vi "load_xml.vi"(8 "error in":errorcluster, 10 "child node in":refnum<k20>, 11 "Hamamatsu_C9100-13.lvclass (in)":refnum<class "Hamamatsu_C9100-13.lvclass">) -> (0 "error out":errorcluster, 2 "child node out":refnum<k20>, 3 "Hamamatsu_C9100-13.lvclass":refnum<class "Hamamatsu_C9100-13.lvclass">)   [LabVIEW 2014, in "Hamamatsu_C9100-13.lvclass"]
doc: "Loads Hamamatsu C9100-13 camera settings from xml. Expected format:\n\n<Enable>%b</Enable>\n<AnalogGain>%u</AnalogGain>\n<FrameGrabberAcquisitionRegion columns=\"left, top, right, bottom\">%u %u %u %u</FrameGrabberAcquisitionRegion>\n<ExposureTime>%f</ExposureTime>\n<EMGain>%u</EMGain>\n<TriggerPolarity>%s</TriggerPolarity>\n<ExternalTriggerMode>%s</ExternalTriggerMode>\n<ScanSpeed>%s</ScanSpeed>\n<ExternalTriggerSource>%s</ExternalTriggerSource>\n<ScanMode>%s</ScanMode>\n<SuperPixelBinning>%s</SuperPixelBinning>\n<CameraSubArrayAcquisitionRegion columns=\"left, top, width, height\">%u %u %u %u</CameraSubArrayAcquisitionRegion>\n<NumberOfImageBuffers>%u</NumberOfImageBuffers>\n<RegionsOfInterest columns=\"Left, Top, Right Bottom\">\n%s</RegionsOfInterest>\n<BackgroundRegions columns=\"Left, Top, Right Bottom\">\n%s</BackgroundRegions>\n<ShotsPerMeasurement>%u</ShotsPerMeasurement>\n<PhotoelectronScaling>%f</PhotoelectronScaling>\n\nMTL 2013 Jan 1"
uses:
  Hamamatsu_C9100-13.lvclass
  Hamamatsu_C9100-13.lvclass/Hamamatsu_C9100-13.ctl
  Globals.vi
  <vilib>/xml/Close Reference(Node).vi
  <resource>/objmgr/DOMUserDefRef.rc
  <vilib>/xml/NI_XML.lvlib
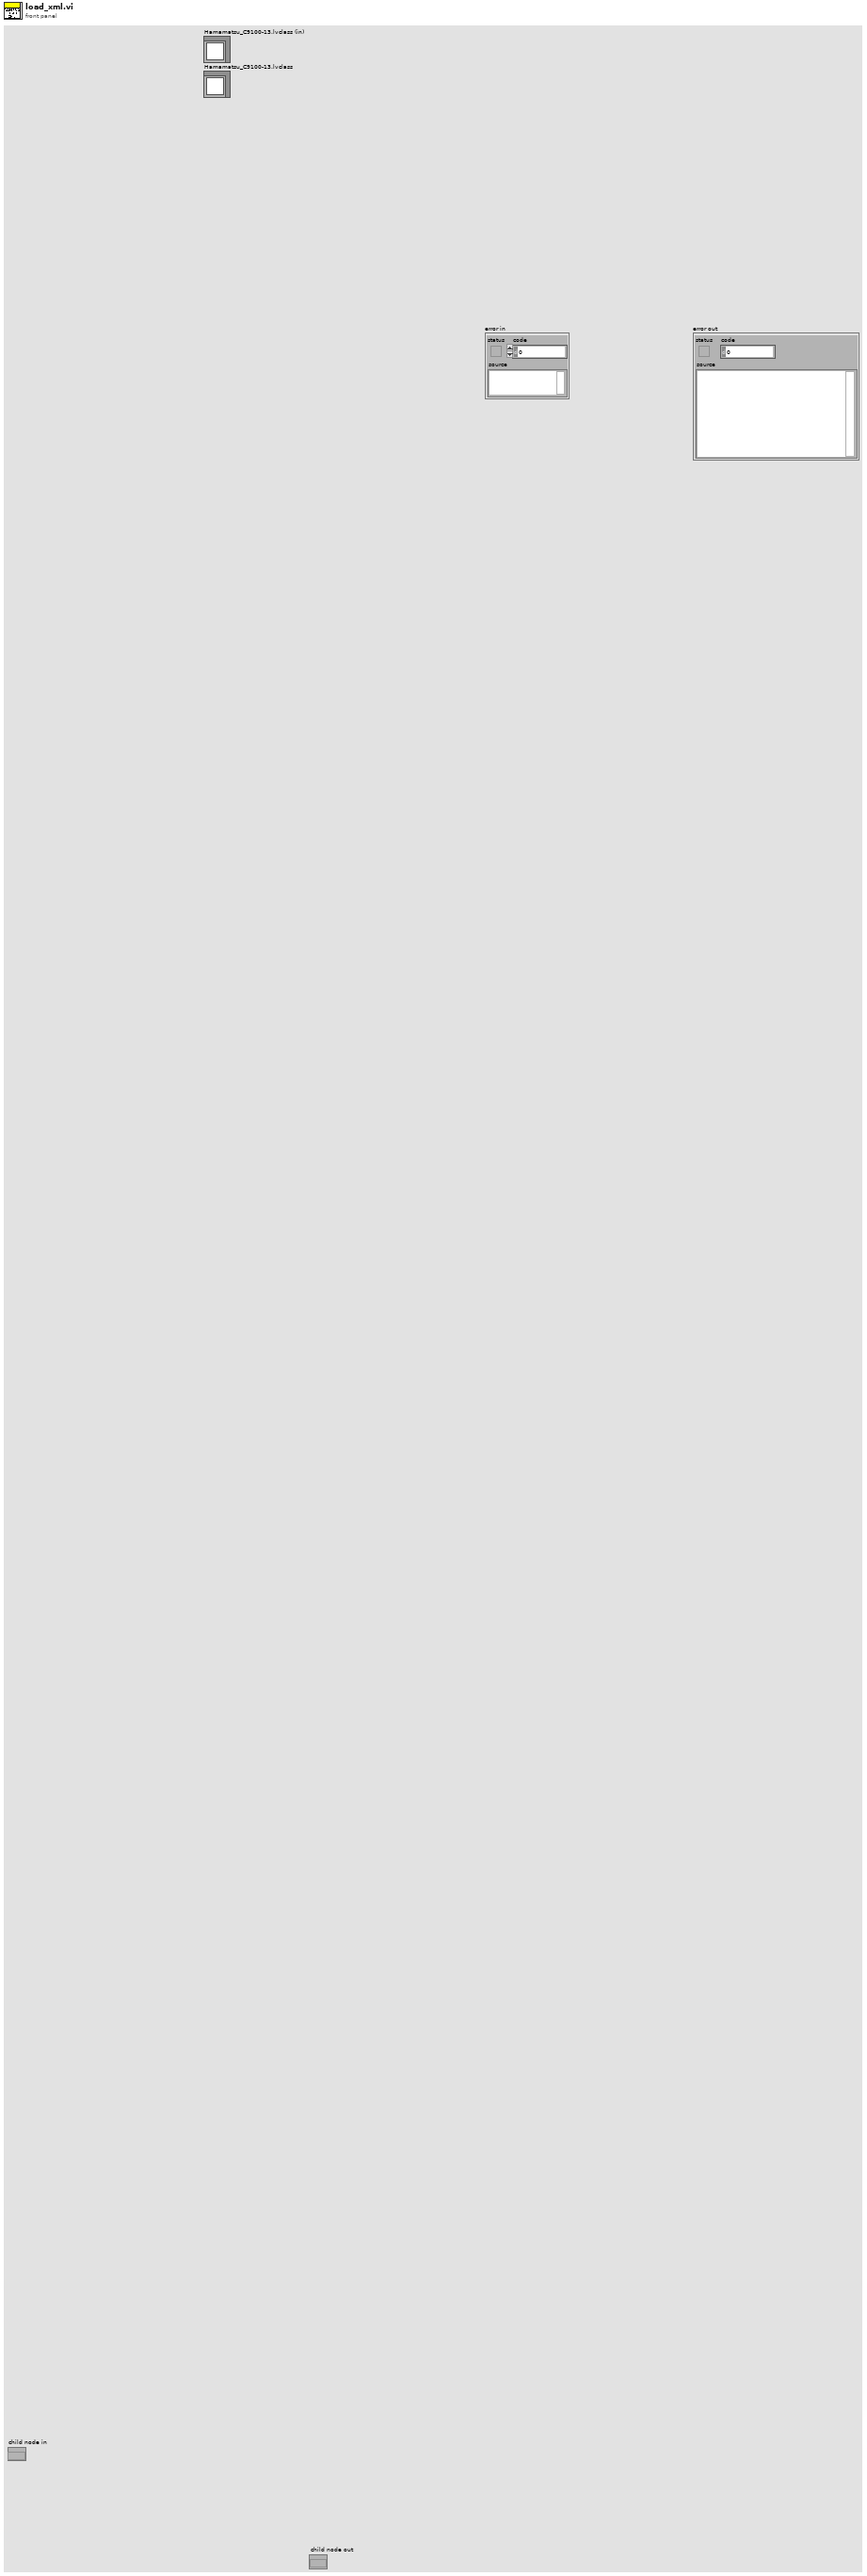
[diagram p1: front panel]
types:
  T1 = typedef "Hamamatsu_C9100-13.lvclass/camera_setup.ctl" = cluster{"Analog Gain (0-5)":u8, "Exposure Time":dbl, "EM Gain (0-255)":u8, "Trigger Polarity":string, "External Trigger Mode":string, "Scan Speed":string, "External Trigger Source":string, "Scan Mode":string, "Super Pixel Binning\n(if enabled in Scan Mode)":string, "Camera Sub-array acquisition region\n(if enabled in scan mode)":cluster{"Left":u16, "Top":u16, "Width":u16, "Height":u16}, "Use camera?":bool, "# image buffers":i32, "shots per measurement":i32, "Force images to U16":bool, "Low Light Sensitivity":string, "cooling":string, "fan":string, "Frame Grabber acquisition region":cluster{"Left":i32, "Top":i32, "Right":i32, "Bottom":i32}}
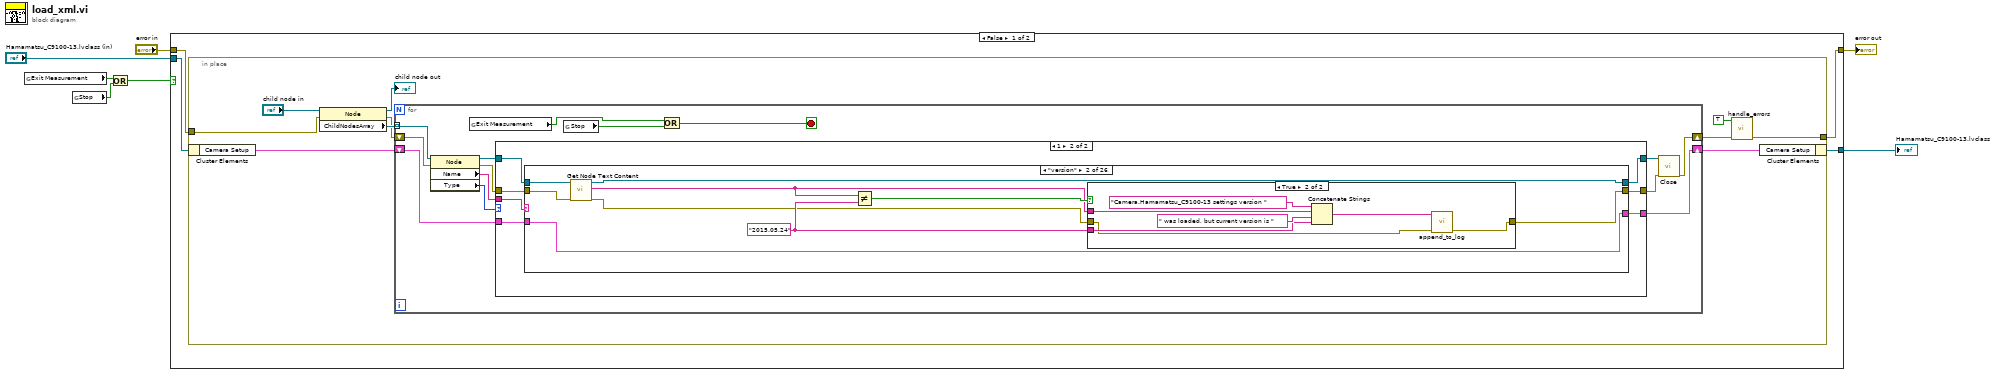
[diagram p0: block diagram]
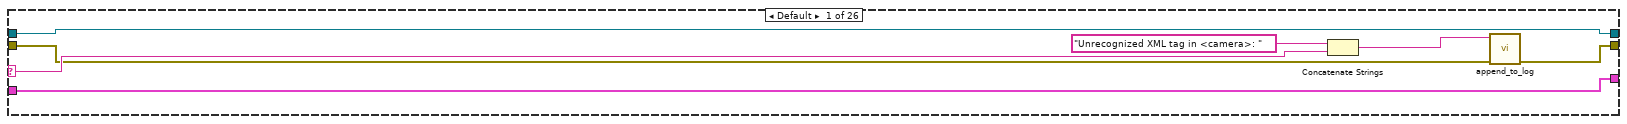
[diagram p3: hidden frame]
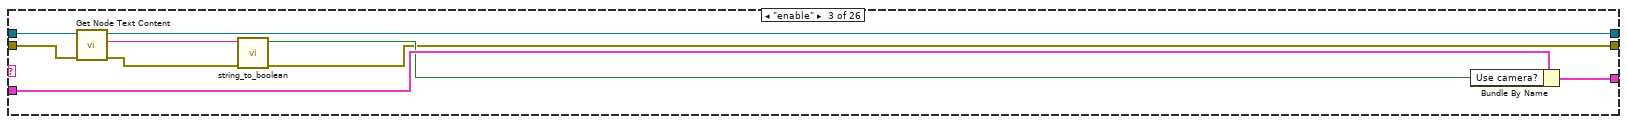
[diagram p5: hidden frame]
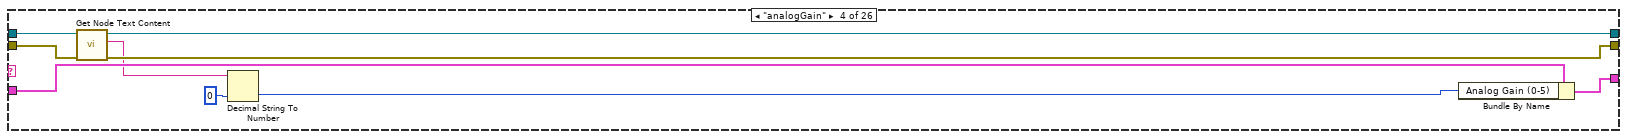
[diagram p6: hidden frame]
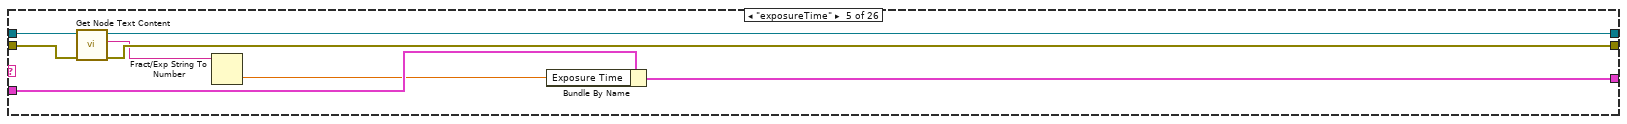
[diagram p7: hidden frame]
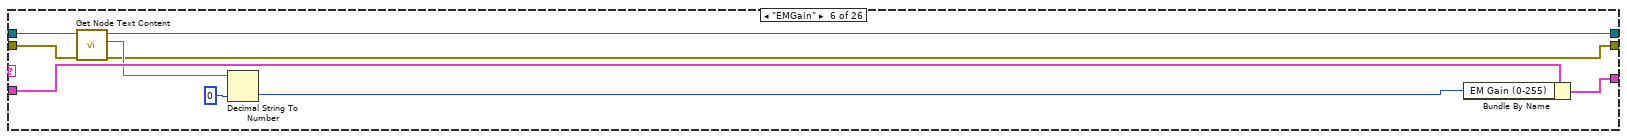
[diagram p8: hidden frame]
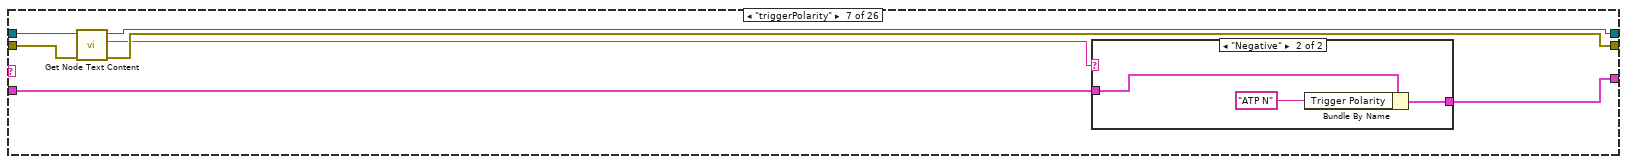
[diagram p9: hidden frame]
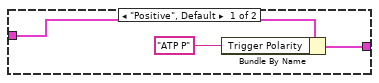
[diagram p10: hidden frame]
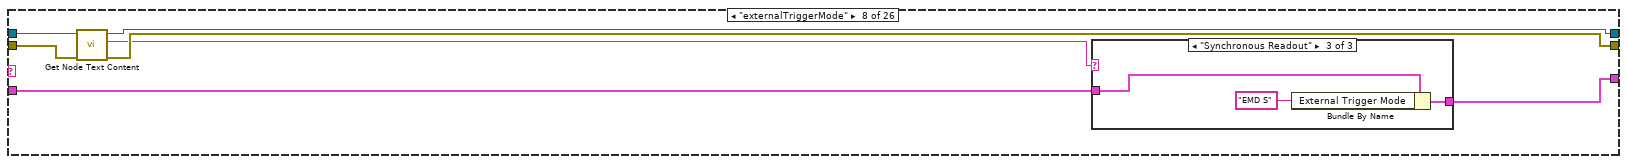
[diagram p11: hidden frame]
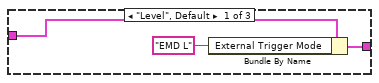
[diagram p12: hidden frame]
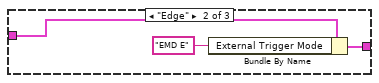
[diagram p13: hidden frame]
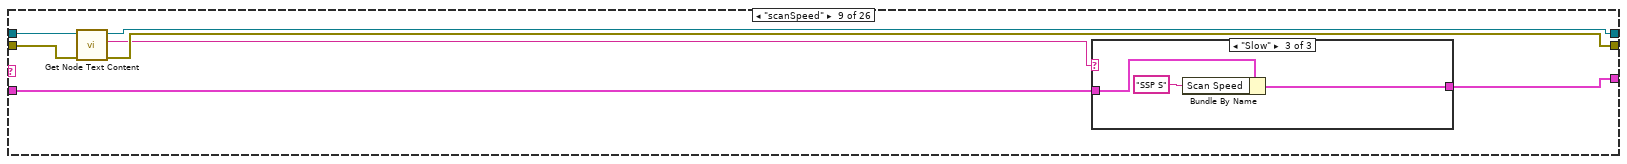
[diagram p14: hidden frame]
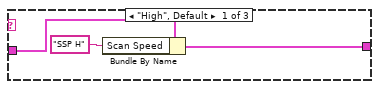
[diagram p15: hidden frame]
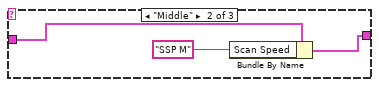
[diagram p16: hidden frame]
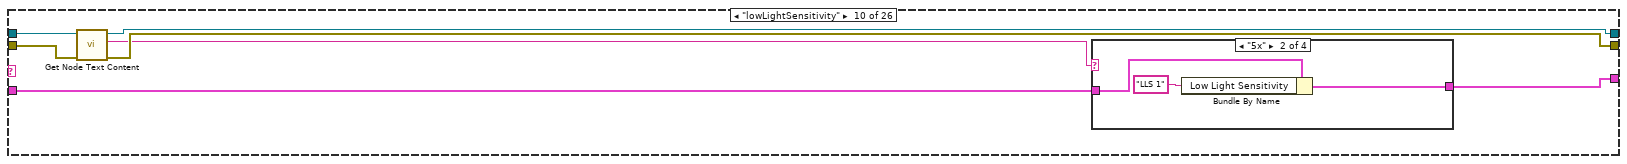
[diagram p17: hidden frame]
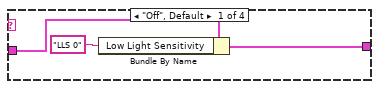
[diagram p18: hidden frame]
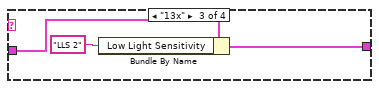
[diagram p19: hidden frame]
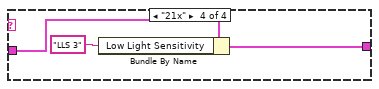
[diagram p20: hidden frame]
diagram:
  n1 = global read "Globals.vi" "Exit Measurement"() -> (w6:bool)
  n2 = global read "Globals.vi" "Stop"() -> (w5:bool)
  n3 = Or(x=w6, y=w5) -> (x .or. y?=w4:bool)
  n4 = case shown="False" w4 {
    tunnel: [w8 w334] -> w7
    tunnel: "error in" -> [w11 w334]
    tunnel: "Hamamatsu_C9100-13.lvclass (in)" -> [w10 w333]
    tunnel: [w9 w333] -> w1
    frame False {
      n5 = in-place {
        in-place-border: [w16] -> w8
        in-place-border: w11 -> [w15]
        n6 = in-place-cluster #1(w10) -> ("Camera Setup"=w13:T1)
        n7 = property class="Node"(reference="child node in", error in=w15) -> (reference out=→"child node out":refnum<k20>, error out=w19:errorcluster, "ChildNodesArray"=w21:refnum<k20>[])
        n8 = for {
          tunnel: w21 -> [w26] mode=indexing
          shift-right: [w32] -> w14
          shift-left: w13 -> [w33]
          shift-right: [w29] -> w17
          shift-left: w19 -> [w27]
          stop <- w22 stop-if-true
          n9 = property class="Node"(reference=w26, error in=w27) -> (reference out=w34:refnum<k20>, error out=w30:errorcluster, "Name"=w35:string, "Type"=w25:i32)
          n10 = global read "Globals.vi" "Exit Measurement"() -> (w24:bool)
          n11 = case shown="1" w25 {
            tunnel: w35 -> [_ w45]
            tunnel: w34 -> [w38 w44]
            tunnel: w33 -> [w36 w43]
            tunnel: [w36 w42] -> w32
            tunnel: [w38 w41] -> w31
            tunnel: w30 -> [w37 w40]
            tunnel: [w37 w39] -> w28
            frame Default {
            }
            frame 1 {
              n12 = case shown="\"version\"" w45 {
                selector: w45 -> [w48 _ _ _ _ _ _ _ _ _ _ _ _ _ _ _ _ _ _ _ _ _ _ _ _ _]
                tunnel: w44 -> [w51 w56 w77 w84 w92 w103 w110 w123 w139 w155 w174 w190 w203 w216 w230 w241 w250 w259 w268 w277 w286 w295 w304 w313 w322 w331]
                tunnel: w43 -> [w52 w55 w75 w87 w95 w101 w107 w120 w136 w152 w171 w187 w199 w213 w233 w238 w247 w256 w265 w274 w283 w292 w301 w311 w320 w324]
                tunnel: [w52 w55 w74 w86 w94 w100 w106 w119 w135 w151 w170 w186 w198 w212 w232 w234 w243 w252 w261 w270 w279 w288 w297 w310 w319 w329] -> w42
                tunnel: [w51 w54 w78 w85 w93 w104 w111 w124 w140 w156 w175 w191 w204 w217 w231 w239 w248 w257 w266 w275 w284 w293 w302 w314 w323 w332] -> w41
                tunnel: w40 -> [w47 w57 w76 w83 w91 w102 w109 w122 w138 w154 w173 w189 w202 w215 w229 w242 w251 w260 w269 w278 w287 w296 w305 w312 w321 w330]
                tunnel: [w46 w53 w70 w82 w90 w98 w108 w121 w137 w153 w172 w188 w201 w214 w228 w240 w249 w258 w267 w276 w285 w294 w303 w308 w317 w327] -> w39
                frame Default {
                  n13 = Concatenate Strings("Unrecognized XML tag in <camera>: " ("string"), w48) -> (w49:string)
                  n14 = call "append_to_log.vi"("error in"=w47, "string"=w49) -> ("error out"=w46:errorcluster)  [unwired: 9 in]
                }
                frame "version" {
                  w59 = "2015.05.24" ("y")
                  n15 = call <vilib>:"Get Node Text Content.vi"("error in (no error)"=w57, "node in"=w56) -> ("error out"=w58:errorcluster, "node text"=w60:string, "node out"=w54:refnum<k20>)  [unwired: 7 in]
                  n16 = Not Equal?(x=w60, y=w59) -> (x != y?=w61:bool)
                  n17 = case shown="True" w61 {
                    tunnel: w60 -> [_ w68]
                    tunnel: w59 -> [_ w66]
                    tunnel: w58 -> [w62 w64]
                    tunnel: [w62 w63] -> w53
                    frame False {
                    }
                    frame True {
                      n18 = Concatenate Strings("Camera.Hamamatsu_C9100-13 settings version " ("string"), w68, " was loaded, but current version is " ("string"), w66) -> (w65:string)
                      n19 = call "append_to_log.vi"("error in"=w64, "string"=w65) -> ("error out"=w63:errorcluster)  [unwired: 9 in]
                    }
                  }
                }
                frame "enable" {
                  n20 = call <vilib>:"Get Node Text Content.vi"("error in (no error)"=w76, "node in"=w77) -> ("error out"=w72:errorcluster, "node text"=w73:string, "node out"=w78:refnum<k20>)  [unwired: 7 in]
                  n21 = call "string_to_boolean.vi"("error in"=w72, "string"=w73) -> ("error out"=w70:errorcluster, "boolean"=w71:bool)  [unwired: 8 in]
                  n22 = Bundle By Name(cluster=w75, "Use camera?"=w71) -> (w74:T1)
                }
                frame "analogGain" {
                  n23 = call <vilib>:"Get Node Text Content.vi"("error in (no error)"=w83, "node in"=w84) -> ("error out"=w82:errorcluster, "node text"=w81:string, "node out"=w85:refnum<k20>)  [unwired: 7 in]
                  n24 = Decimal String To Number(string=w81, default (0L)=u8 0 ("Analog Gain (0-5)")) -> (number=w79:u8)  [unwired: 1 in, 1 out]
                  n25 = Bundle By Name(cluster=w87, "Analog Gain (0-5)"=w79) -> (w86:T1)
                }
                frame "exposureTime" {
                  n26 = call <vilib>:"Get Node Text Content.vi"("error in (no error)"=w91, "node in"=w92) -> ("error out"=w90:errorcluster, "node text"=w89:string, "node out"=w93:refnum<k20>)  [unwired: 7 in]
                  n27 = Fract/Exp String To Number(string=w89) -> (number=w88:dbl)  [unwired: 3 in, 1 out]
                  n28 = Bundle By Name(cluster=w95, "Exposure Time"=w88) -> (w94:T1)
                }
                frame "EMGain" {
                  n29 = call <vilib>:"Get Node Text Content.vi"("error in (no error)"=w102, "node in"=w103) -> ("error out"=w98:errorcluster, "node text"=w99:string, "node out"=w104:refnum<k20>)  [unwired: 7 in]
                  n30 = Decimal String To Number(string=w99, default (0L)=u8 0 ("EM Gain (0-255)")) -> (number=w96:u8)  [unwired: 1 in, 1 out]
                  n31 = Bundle By Name(cluster=w101, "EM Gain (0-255)"=w96) -> (w100:T1)
                }
                frame "triggerPolarity" {
                  n32 = call <vilib>:"Get Node Text Content.vi"("error in (no error)"=w109, "node in"=w110) -> ("error out"=w108:errorcluster, "node text"=w105:string, "node out"=w111:refnum<k20>)  [unwired: 7 in]
                  n33 = case shown="\"Negative\"" w105 {
                    tunnel: w107 -> [w114 w117]
                    tunnel: [w113 w116] -> w106
                    frame "Positive", Default {
                      n34 = Bundle By Name(cluster=w114, "Trigger Polarity"="ATP P" ("fan")) -> (w113:T1)
                    }
                    frame "Negative" {
                      n35 = Bundle By Name(cluster=w117, "Trigger Polarity"="ATP N" ("fan")) -> (w116:T1)
                    }
                  }
                }
                frame "externalTriggerMode" {
                  n36 = call <vilib>:"Get Node Text Content.vi"("error in (no error)"=w122, "node in"=w123) -> ("error out"=w121:errorcluster, "node text"=w118:string, "node out"=w124:refnum<k20>)  [unwired: 7 in]
                  n37 = case shown="\"Synchronous Readout\"" w118 {
                    tunnel: w120 -> [w127 w130 w133]
                    tunnel: [w126 w129 w132] -> w119
                    frame "Level", Default {
                      n38 = Bundle By Name(cluster=w127, "External Trigger Mode"="EMD L" ("fan")) -> (w126:T1)
                    }
                    frame "Edge" {
                      n39 = Bundle By Name(cluster=w130, "External Trigger Mode"="EMD E" ("fan")) -> (w129:T1)
                    }
                    frame "Synchronous Readout" {
                      n40 = Bundle By Name(cluster=w133, "External Trigger Mode"="EMD S" ("fan")) -> (w132:T1)
                    }
                  }
                }
                frame "scanSpeed" {
                  n41 = call <vilib>:"Get Node Text Content.vi"("error in (no error)"=w138, "node in"=w139) -> ("error out"=w137:errorcluster, "node text"=w134:string, "node out"=w140:refnum<k20>)  [unwired: 7 in]
                  n42 = case shown="\"Slow\"" w134 {
                    tunnel: w136 -> [w143 w146 w149]
                    tunnel: [w142 w145 w148] -> w135
                    frame "High", Default {
                      n43 = Bundle By Name(cluster=w143, "Scan Speed"="SSP H" ("fan")) -> (w142:T1)
                    }
                    frame "Middle" {
                      n44 = Bundle By Name(cluster=w146, "Scan Speed"="SSP M" ("fan")) -> (w145:T1)
                    }
                    frame "Slow" {
                      n45 = Bundle By Name(cluster=w149, "Scan Speed"="SSP S" ("fan")) -> (w148:T1)
                    }
                  }
                }
                frame "lowLightSensitivity" {
                  n46 = call <vilib>:"Get Node Text Content.vi"("error in (no error)"=w154, "node in"=w155) -> ("error out"=w153:errorcluster, "node text"=w150:string, "node out"=w156:refnum<k20>)  [unwired: 7 in]
                  n47 = case shown="\"5x\"" w150 {
                    tunnel: w152 -> [w159 w162 w165 w168]
                    tunnel: [w158 w161 w164 w167] -> w151
                    frame "Off", Default {
                      n48 = Bundle By Name(cluster=w159, "Low Light Sensitivity"="LLS 0" ("fan")) -> (w158:T1)
                    }
                    frame "5x" {
                      n49 = Bundle By Name(cluster=w162, "Low Light Sensitivity"="LLS 1" ("fan")) -> (w161:T1)
                    }
                    frame "13x" {
                      n50 = Bundle By Name(cluster=w165, "Low Light Sensitivity"="LLS 2" ("fan")) -> (w164:T1)
                    }
                    frame "21x" {
                      n51 = Bundle By Name(cluster=w168, "Low Light Sensitivity"="LLS 3" ("fan")) -> (w167:T1)
                    }
                  }
                }
                frame "externalTriggerSource" {
                  n52 = call <vilib>:"Get Node Text Content.vi"("error in (no error)"=w173, "node in"=w174) -> ("error out"=w172:errorcluster, "node text"=w169:string, "node out"=w175:refnum<k20>)  [unwired: 7 in]
                  n53 = case shown="\"CameraLink Interface\"" w169 {
                    tunnel: w171 -> [w178 w181 w184]
                    tunnel: [w177 w180 w183] -> w170
                    frame "Multi-Timing I/O Pin" {
                      n54 = Bundle By Name(cluster=w178, "External Trigger Source"="ESC M" ("fan")) -> (w177:T1)
                    }
                    frame "BNC on Power Supply", Default {
                      n55 = Bundle By Name(cluster=w181, "External Trigger Source"="ESC B" ("fan")) -> (w180:T1)
                    }
                    frame "CameraLink Interface" {
                      n56 = Bundle By Name(cluster=w184, "External Trigger Source"="ESC I" ("fan")) -> (w183:T1)
                    }
                  }
                }
                frame "cooling" {
                  n57 = call <vilib>:"Get Node Text Content.vi"("error in (no error)"=w189, "node in"=w190) -> ("error out"=w188:errorcluster, "node text"=w185:string, "node out"=w191:refnum<k20>)  [unwired: 7 in]
                  n58 = case shown="\"On\"" w185 {
                    tunnel: w187 -> [w194 w197]
                    tunnel: [w193 w196] -> w186
                    frame "On" {
                      n59 = Bundle By Name(cluster=w194, "cooling"="CSW O" ("fan")) -> (w193:T1)
                    }
                    frame "Off", Default {
                      n60 = Bundle By Name(cluster=w197, "cooling"="CSW F" ("fan")) -> (w196:T1)
                    }
                  }
                }
                frame "fan" {
                  n61 = call <vilib>:"Get Node Text Content.vi"("error in (no error)"=w202, "node in"=w203) -> ("error out"=w201:errorcluster, "node text"=w200:string, "node out"=w204:refnum<k20>)  [unwired: 7 in]
                  n62 = case shown="\"Off\", Default" w200 {
                    tunnel: w199 -> [w207 w210]
                    tunnel: [w206 w209] -> w198
                    frame "On" {
                      n63 = Bundle By Name(cluster=w207, "fan"="FAN O") -> (w206:T1)
                    }
                    frame "Off", Default {
                      n64 = Bundle By Name(cluster=w210, "fan"="FAN F") -> (w209:T1)
                    }
                  }
                }
                frame "scanMode" {
                  n65 = call <vilib>:"Get Node Text Content.vi"("error in (no error)"=w215, "node in"=w216) -> ("error out"=w214:errorcluster, "node text"=w211:string, "node out"=w217:refnum<k20>)  [unwired: 7 in]
                  n66 = case shown="\"Sub-array\"" w211 {
                    tunnel: w213 -> [w220 w223 w226]
                    tunnel: [w219 w222 w225] -> w212
                    frame "Normal", Default {
                      n67 = Bundle By Name(cluster=w220, "Scan Mode"="SMD N" ("fan")) -> (w219:T1)
                    }
                    frame "Super Pixel" {
                      n68 = Bundle By Name(cluster=w223, "Scan Mode"="SMD S" ("fan")) -> (w222:T1)
                    }
                    frame "Sub-array" {
                      n69 = Bundle By Name(cluster=w226, "Scan Mode"="SMD A" ("fan")) -> (w225:T1)
                    }
                  }
                }
                frame "superPixelBinning" {
                  n70 = call <vilib>:"Get Node Text Content.vi"("error in (no error)"=w229, "node in"=w230) -> ("error out"=w228:errorcluster, "node text"=w227:string, "node out"=w231:refnum<k20>)  [unwired: 7 in]
                  n71 = Bundle By Name(cluster=w233, "Super Pixel Binning\n(if enabled in Scan Mode)"=w227) -> (w232:T1)
                }
                frame "subArrayLeft" {
                  n72 = call <vilib>:"Get Node Text Content.vi"("error in (no error)"=w242, "node in"=w241) -> ("error out"=w240:errorcluster, "node text"=w236:string, "node out"=w239:refnum<k20>)  [unwired: 7 in]
                  n73 = Decimal String To Number(string=w236, default (0L)=u16 0 ("EM Gain (0-255)")) -> (number=w235:u16)  [unwired: 1 in, 1 out]
                  n74 = Bundle By Name(cluster=w238, "Camera Sub-array acquisition region\n(if enabled in scan mode).Left"=w235) -> (w234:T1)
                }
                frame "subArrayTop" {
                  n75 = call <vilib>:"Get Node Text Content.vi"("error in (no error)"=w251, "node in"=w250) -> ("error out"=w249:errorcluster, "node text"=w245:string, "node out"=w248:refnum<k20>)  [unwired: 7 in]
                  n76 = Decimal String To Number(string=w245, default (0L)=u16 0 ("EM Gain (0-255)")) -> (number=w244:u16)  [unwired: 1 in, 1 out]
                  n77 = Bundle By Name(cluster=w247, "Camera Sub-array acquisition region\n(if enabled in scan mode).Top"=w244) -> (w243:T1)
                }
                frame "subArrayWidth" {
                  n78 = call <vilib>:"Get Node Text Content.vi"("error in (no error)"=w260, "node in"=w259) -> ("error out"=w258:errorcluster, "node text"=w254:string, "node out"=w257:refnum<k20>)  [unwired: 7 in]
                  n79 = Decimal String To Number(string=w254, default (0L)=u16 0 ("EM Gain (0-255)")) -> (number=w253:u16)  [unwired: 1 in, 1 out]
                  n80 = Bundle By Name(cluster=w256, "Camera Sub-array acquisition region\n(if enabled in scan mode).Width"=w253) -> (w252:T1)
                }
                frame "subArrayHeight" {
                  n81 = call <vilib>:"Get Node Text Content.vi"("error in (no error)"=w269, "node in"=w268) -> ("error out"=w267:errorcluster, "node text"=w263:string, "node out"=w266:refnum<k20>)  [unwired: 7 in]
                  n82 = Decimal String To Number(string=w263, default (0L)=u16 0 ("EM Gain (0-255)")) -> (number=w262:u16)  [unwired: 1 in, 1 out]
                  n83 = Bundle By Name(cluster=w265, "Camera Sub-array acquisition region\n(if enabled in scan mode).Height"=w262) -> (w261:T1)
                }
                frame "frameGrabberAcquisitionRegionLeft" {
                  n84 = call <vilib>:"Get Node Text Content.vi"("error in (no error)"=w278, "node in"=w277) -> ("error out"=w276:errorcluster, "node text"=w272:string, "node out"=w275:refnum<k20>)  [unwired: 7 in]
                  n85 = Decimal String To Number(string=w272, default (0L)=0 ("EM Gain (0-255)")) -> (number=w271:i32)  [unwired: 1 in, 1 out]
                  n86 = Bundle By Name(cluster=w274, "Frame Grabber acquisition region.Left"=w271) -> (w270:T1)
                }
                frame "frameGrabberAcquisitionRegionTop" {
                  n87 = call <vilib>:"Get Node Text Content.vi"("error in (no error)"=w287, "node in"=w286) -> ("error out"=w285:errorcluster, "node text"=w281:string, "node out"=w284:refnum<k20>)  [unwired: 7 in]
                  n88 = Decimal String To Number(string=w281, default (0L)=0 ("EM Gain (0-255)")) -> (number=w280:i32)  [unwired: 1 in, 1 out]
                  n89 = Bundle By Name(cluster=w283, "Frame Grabber acquisition region.Top"=w280) -> (w279:T1)
                }
                frame "frameGrabberAcquisitionRegionRight" {
                  n90 = call <vilib>:"Get Node Text Content.vi"("error in (no error)"=w296, "node in"=w295) -> ("error out"=w294:errorcluster, "node text"=w290:string, "node out"=w293:refnum<k20>)  [unwired: 7 in]
                  n91 = Decimal String To Number(string=w290, default (0L)=0 ("EM Gain (0-255)")) -> (number=w289:i32)  [unwired: 1 in, 1 out]
                  n92 = Bundle By Name(cluster=w292, "Frame Grabber acquisition region.Right"=w289) -> (w288:T1)
                }
                frame "frameGrabberAcquisitionRegionBottom" {
                  n93 = call <vilib>:"Get Node Text Content.vi"("error in (no error)"=w305, "node in"=w304) -> ("error out"=w303:errorcluster, "node text"=w299:string, "node out"=w302:refnum<k20>)  [unwired: 7 in]
                  n94 = Decimal String To Number(string=w299, default (0L)=0 ("EM Gain (0-255)")) -> (number=w298:i32)  [unwired: 1 in, 1 out]
                  n95 = Bundle By Name(cluster=w301, "Frame Grabber acquisition region.Bottom"=w298) -> (w297:T1)
                }
                frame "numImageBuffers" {
                  n96 = call <vilib>:"Get Node Text Content.vi"("error in (no error)"=w312, "node in"=w313) -> ("error out"=w308:errorcluster, "node text"=w309:string, "node out"=w314:refnum<k20>)  [unwired: 7 in]
                  n97 = Decimal String To Number(string=w309, default (0L)=0 ("EM Gain (0-255)")) -> (number=w306:i32)  [unwired: 1 in, 1 out]
                  n98 = Bundle By Name(cluster=w311, "# image buffers"=w306) -> (w310:T1)
                }
                frame "shotsPerMeasurement" {
                  n99 = call <vilib>:"Get Node Text Content.vi"("error in (no error)"=w321, "node in"=w322) -> ("error out"=w317:errorcluster, "node text"=w318:string, "node out"=w323:refnum<k20>)  [unwired: 7 in]
                  n100 = Decimal String To Number(string=w318, default (0L)=0 ("EM Gain (0-255)")) -> (number=w315:i32)  [unwired: 1 in, 1 out]
                  n101 = Bundle By Name(cluster=w320, "shots per measurement"=w315) -> (w319:T1)
                }
                frame "forceImagesToU16" {
                  n102 = call <vilib>:"Get Node Text Content.vi"("error in (no error)"=w330, "node in"=w331) -> ("error out"=w328:errorcluster, "node text"=w326:string, "node out"=w332:refnum<k20>)  [unwired: 7 in]
                  n103 = call "string_to_boolean.vi"("error in"=w328, "string"=w326) -> ("error out"=w327:errorcluster, "boolean"=w325:bool)  [unwired: 8 in]
                  n104 = Bundle By Name(cluster=w324, "Force images to U16"=w325) -> (w329:T1)
                }
              }
            }
          }
          n105 = global read "Globals.vi" "Stop"() -> (w23:bool)
          n106 = Or(x=w24, y=w23) -> (x .or. y?=w22:bool)
          n107 = call-poly <vilib>:"Close.vi"("error in (no error)"=w28, "node"=w31) -> ("error out"=w29:errorcluster)  [unwired: 7 in]
        }
        n108 = call "handle_errors.vi"("Exit Operation"=TRUE, "error in (no error)"=w17) -> ("error out"=w16:errorcluster)  [unwired: 13 in]
        n109 = in-place-cluster #1("Camera Setup"=w14) -> (w9:refnum<class "Hamamatsu_C9100-13.lvclass">)
      }
    }
    frame True {
    }
  }
  "error out" <- w7
  "Hamamatsu_C9100-13.lvclass" <- w1
